vi "niTuner Error Handler.vi"(8 "error in":errorcluster, 9 "pop up message?":bool, 11 "taskID in":i32) -> (0 "error out":errorcluster, 2 "error message":string, 3 "taskID out":i32)   [LabVIEW 2011]
uses:
  nipxi5600u.dll
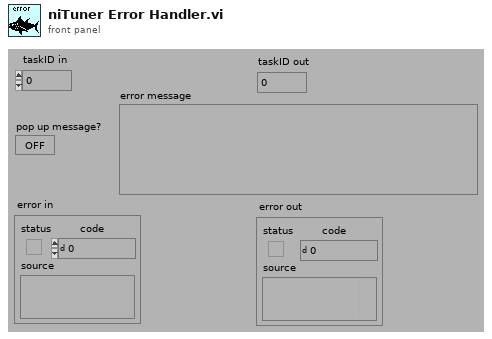
[diagram p1: front panel]
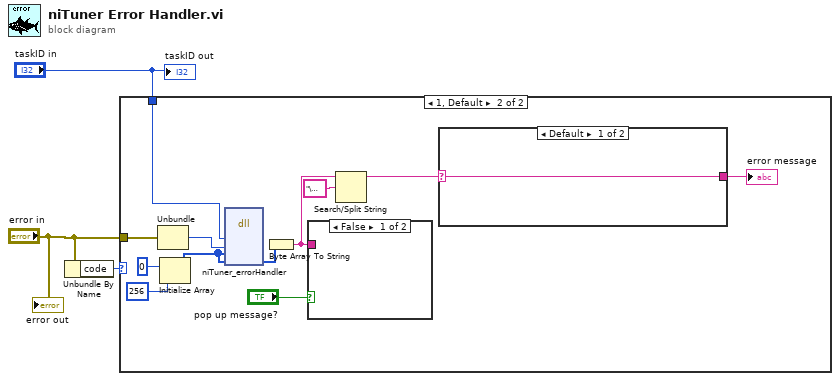
[diagram p0: block diagram]
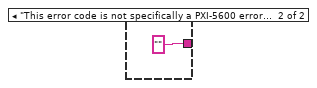
[diagram p3: hidden frame]
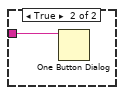
[diagram p4: hidden frame]
diagram:
  n1 = Unbundle By Name("error in") -> ("code"=w1:i32)
  n2 = case shown="1, Default" w1 {
    tunnel: "error in" -> [_ w15]
    tunnel: "taskID in" -> [_ w8]
    frame 0 {
    }
    frame 1, Default {
      n3 = Unbundle(w15) -> ("code"=w9:i32)  [unwired: 2 out]
      n4 = Initialize Array(u8 0, 256 ("Dimension Size")) -> (w11:u8[])
      n5 = dll-call lib="nipxi5600u.dll" fn="niTuner_errorHandler"("taskID"=w8, "errorCode"=w9, "errorSource"=w11, "errorDescription"=w11) -> ("errorDescription"=w10:u8[])  [unwired: 7 in, 2 out]
      n6 = Byte Array To String(unsigned byte array=w10) -> (string=w7:string)
      n7 = case shown="False" "pop up message?" {
        tunnel: w7 -> [_ w18]
        frame False {
        }
        frame True {
          n8 = One Button Dialog(message=w18) -> ()  [unwired: 1 in, 1 out]
        }
      }
      n9 = Search/Split String(string=w7, search string/char (-)="\u0000") -> (substring before match=w5:string)  [unwired: 1 in, 2 out]
      n10 = case shown="Default" w5 {
        selector: w5 -> [w16 _]
        tunnel: [w16 "" ("error message")] -> w4
        frame Default {
        }
        frame "This error code is not specifically a PXI-5600 error" {
        }
      }
      "error message" <- w4
    }
  }
  "error out" <- "error in"
  "taskID out" <- "taskID in"
